vi "VI-Grow Nodes.vi"(2 "Components":T1, 9 "Numeric":i32, 11 "error in (no error)":errorcluster) -> (15 "error out":errorcluster)   [LabVIEW 2015]
uses:
  VI-Reg Event Components.ctl
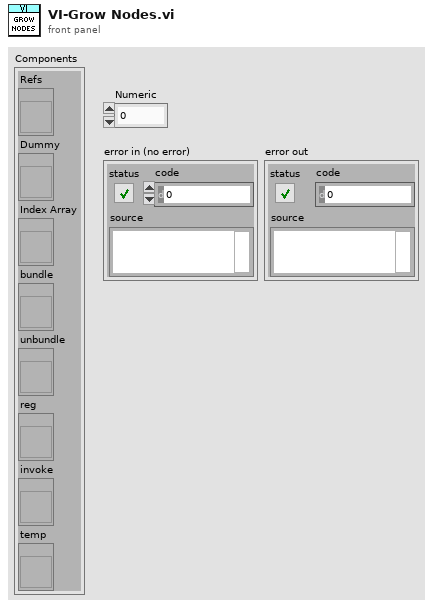
[diagram p1: front panel]
types:
  T1 = typedef "VI-Reg Event Components.ctl" = cluster{"Refs":refnum<vi>, "Dummy":refnum<vi>, "Index Array":refnum<vi>, "bundle":refnum<vi>, "unbundle":refnum<vi>, "reg":refnum<vi>, "invoke":refnum<vi>, "temp":refnum<vi>}
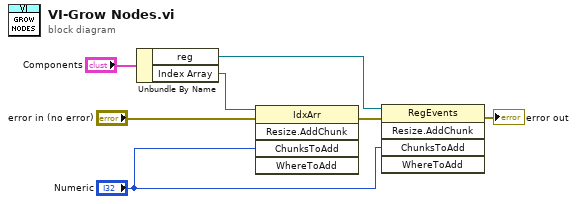
[diagram p0: block diagram]
diagram:
  n1 = Unbundle By Name("Components") -> ("reg"=w7:refnum<vi>, "Index Array"=w5:refnum<vi>)
  n2 = invoke class="IdxArr" method="Resize.AddChunk"(reference=w5, error in="error in (no error)", "ChunksToAdd"="Numeric") -> (error out=w6:errorcluster)  [unwired: 2 in, 4 out]
  n3 = invoke class="RegEvents" method="Resize.AddChunk"(reference=w7, error in=w6, "ChunksToAdd"="Numeric") -> (error out=→"error out":errorcluster)  [unwired: 2 in, 4 out]
